vi "Util String Simplified.vi"(8 "error in (no error)":errorcluster, 11 "String Input":string) -> (0 "error out":errorcluster, 3 "String Output":string)   [LabVIEW 2017, in "xHelper.lvlib"]
uses:
  xHelper.lvlib
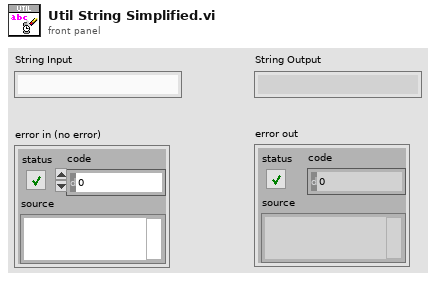
[diagram p1: front panel]
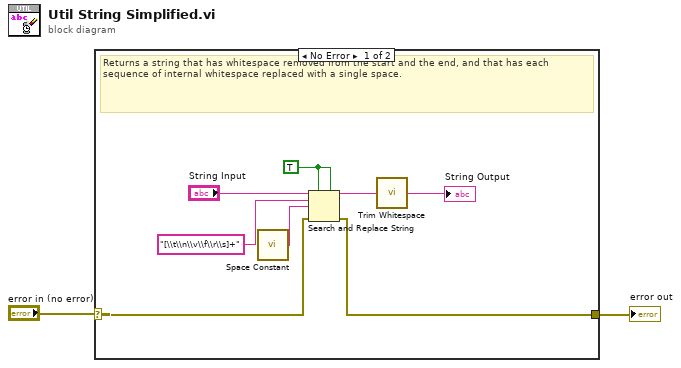
[diagram p0: block diagram]
diagram:
  n1 = case shown="No Error" "error in (no error)" {
    selector: "error in (no error)" -> [w6 w11]
    tunnel: [w5 w11] -> w1
    frame No Error {
      w10 = TRUE ("replace all? (F)")
      # "Returns a string that has whitespace removed from the start and the end, and that has each sequence of internal whitespace replaced with a single space."
      n2 = call <vilib>:"Space Constant.vi"() -> ("String"=w7:string)
      n3 = Search and Replace String(replace all?=w10, multiline?=w10, input string="String Input", search string="[\\t\\n\\v\\f\\r\\s]+" ("replace string (\"\")"), replace string=w7, error in=w6) -> (result string=w4:string, error out=w5:errorcluster)  [unwired: 2 in, 2 out]
      n4 = call <vilib>:"Trim Whitespace.vi"("string"=w4) -> ("trimmed string"=→"String Output":string)  [unwired: 1 in]
    }
    frame Error {
    }
  }
  "error out" <- w1
